vi "Deviation.vi"(11 "2D  Array":u64[][](array[numeric])) -> (0 "Deviation by row":i64[][](array[numeric]), 3 "Average in row":u64[](array[numeric]) format="%-2.0f")   [LabVIEW 2023]
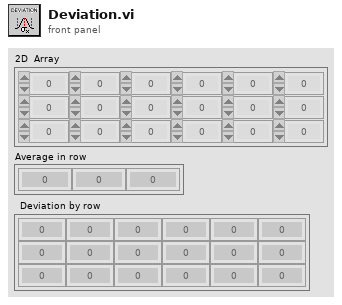
[diagram p1: front panel]
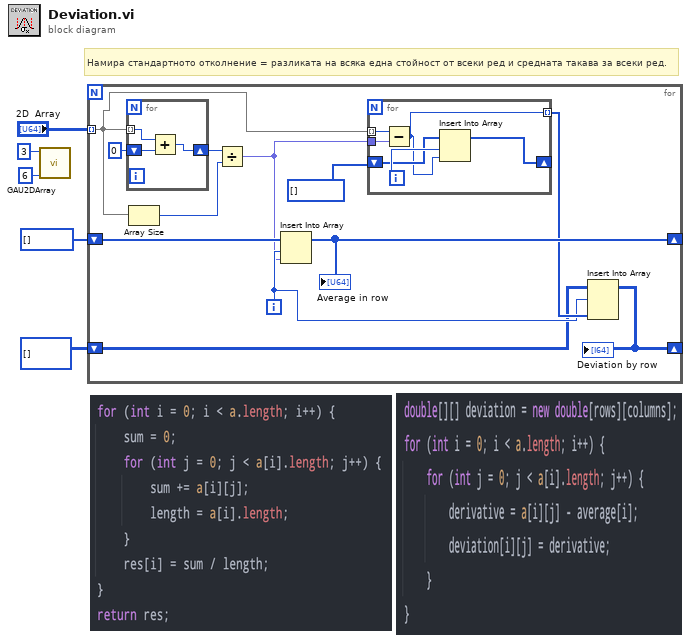
[diagram p0: block diagram]
diagram:
  # "Намира стандартното отколнение = разликата на всяка една стойност от всеки ред и средната такава за всеки ред."
  n1 = call "GAU2DArray.vi"("Colums"=6, "Rows"=3) -> ()  [unwired: 8 in, 2 out]
  n2 = for {
    tunnel: "2D  Array" -> [w12] mode=indexing
    shift-right: [w11] -> _
    shift-left: u64[] [] -> [w15]
    shift-right: [w6] -> _
    shift-left: i64[][] [] -> [w8]
    i -> [w9]
    n3 = for {
      tunnel: w12 -> [w26] mode=indexing
      shift-right: [w25] -> w14
      shift-left: 0 -> [w24]
      n4 = Add(x=w26, y=w24) -> (x+y=w25:u64)
    }
    n5 = Array Size(array=w12) -> (size(s)=w16:i32)
    n6 = Divide(x=w14, y=w16) -> (x/y=w7:fxp<+/-,32,16>)
    n7 = Insert Into Array "Insert Into Array"(array=w15, index=w9, new element=w7) -> (w11:u64[])
    "Average in row" <- w11
    n8 = for {
      tunnel: w12 -> [w23] mode=indexing
      tunnel: w7 -> [w22]
      shift-right: [w19] -> _
      shift-left: u64[] [] -> [w20]
      tunnel: [w18] -> w10 mode=indexing
      i -> [w21]
      n9 = Subtract(x=w23, y=w22) -> (x-y=w18:i64)
      n10 = Insert Into Array(array=w20, index=w21, new element=w18) -> (w19:u64[])
    }
    n11 = Insert Into Array "Insert Into Array"(array=w8, index (row)=w9, new element=w10) -> (w6:i64[][])  [unwired: 1 in]
    "Deviation by row" <- w6
  }
